vi "Get Wave.vi"(8 "error in (no error)":errorcluster, 11 "MIDI Controls in":T1=variant(dbl 0.0)) -> (0 "error out":errorcluster, 2 "Instrument Level Processing out":T2, 3 "MIDI Controls":T1=variant(dbl 0.0))   [LabVIEW 2014, in "mySynthesizer.lvlib"]
uses:
  mySynthesizer.lvlib
  Instrument Level Processing/Instrument Level Processing.ctl
  MIDI Controls/MIDI Controls.ctl
  Signal Generation/Signal Generation.lvlib
  Voice Level Processing/Voice Level Processing.lvlib
  Instrument Level Controls/Instrument Level Controls.lvlib
  Instrument Level Processing/Instrument Level Processing.lvlib
  Voice Level Controls/Voice Level Controls.lvlib
  MIDI Controls/MIDI Controls.lvlib
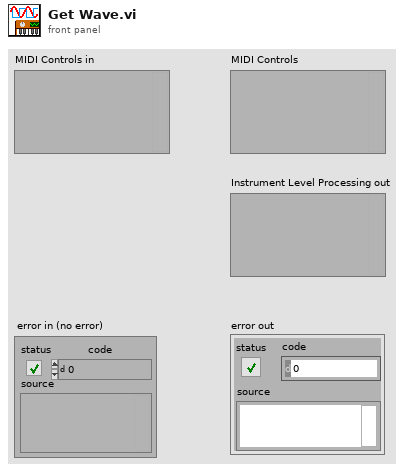
[diagram p1: front panel]
types:
  T1 = typedef "mySynthesizer.lvlib/MIDI Controls.lvlib/MIDI Controls.ctl" = variant
  T2 = typedef "mySynthesizer.lvlib/Instrument Level Processing.lvlib/Instrument Level Processing.ctl" = variant
  T3 = typedef "mySynthesizer.lvlib/Voice Level Controls.lvlib/Voice Level Controls.ctl" = variant
  T4 = typedef "mySynthesizer.lvlib/Instrument Level Controls.lvlib/Instrument Level Controls.ctl" = variant
  T5 = typedef "mySynthesizer.lvlib/Signal Generation.lvlib/Signal Generation Control.ctl" = variant
  T6 = typedef "mySynthesizer.lvlib/Voice Level Processing.lvlib/Voice Level Processing.ctl" = variant
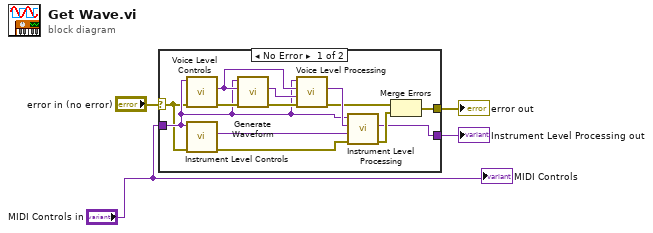
[diagram p0: block diagram]
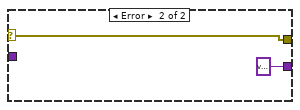
[diagram p2: hidden frame]
diagram:
  n1 = case shown="No Error" "error in (no error)" {
    selector: "error in (no error)" -> [w5 w18]
    tunnel: [w8 w18] -> w4
    tunnel: [w7 variant ("Instrument Level Processing out")] -> w3
    tunnel: "MIDI Controls in" -> [w6 _]
    frame No Error {
      n2 = call "Voice Level Controls.vi"("error in"=w5, "MIDI Controls in"=w6) -> ("error out"=w12:errorcluster, "Voice Level Controls out"=w14:T3)  [unwired: 8 in]
      n3 = call "Instrument Level Controls.vi"("error in (no error)"=w5, "MIDI Controls in"=w6) -> ("error out"=w11:errorcluster, "Instrument Level Controls out"=w15:T4)  [unwired: 8 in]
      n4 = call "Generate Waveform.vi"("error in (no error)"=w12, "Voice Level Controls in"=w14, "MIDI Controls in"=w6) -> ("error out"=w13:errorcluster, "Signal Generation out"=w17:T5)  [unwired: 7 in]
      n5 = call "Voice Level Processing.vi"("error in (no error)"=w13, "Signal Generation in"=w17, "Voice Level Controls in"=w14, "MIDI Controls in"=w6) -> ("error out"=w9:errorcluster, "Voice Level Processing out"=w16:T6)  [unwired: 6 in]
      n6 = call "Instrument Level Processing.vi"("error in (no error)"=w11, "Instrument Level Controls in"=w15, "Voice Level Processing in"=w16, "MIDI Controls in"=w6) -> ("error out"=w10:errorcluster, "Instrument Level Processing out"=w7:T2)  [unwired: 6 in]
      n7 = Merge Errors(w9, w10) -> (w8:errorcluster)
    }
    frame Error {
    }
  }
  "error out" <- w4
  "Instrument Level Processing out" <- w3
  "MIDI Controls" <- "MIDI Controls in"
